vi "destroy_lookup.vi"(8 "error in (no error)":errorcluster, 11 "Lookup Service in":refnum<class "Lookup Service.lvclass">) -> (0 "error out":errorcluster, 1 "remaining references":refnum<data-value>[](array[refnum]))   [LabVIEW 2019, in "Lookup API.lvlib" / "Lookup Service.lvclass"]
uses:
  Lookup Service.lvclass
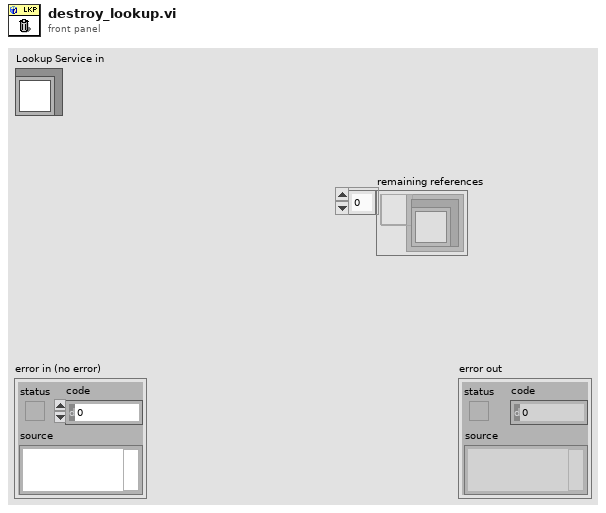
[diagram p1: front panel]
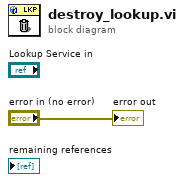
[diagram p0: block diagram]
diagram:
  "error out" <- "error in (no error)"
